vi "CloseConnection.vi"(8 "error in (no error)":errorcluster, 11 "I2COUSBSim in":refnum<class "I2COUSBSim.lvclass">) -> (0 "error out":errorcluster, 1 "Status":string, 3 "I2COUSBSim out":refnum<class "I2COUSBSim.lvclass">)   [LabVIEW 2020, in "I2COUSBSim.lvlib" / "I2COUSBSim.lvclass"]
doc: "Close connection"
uses:
  I2COUSBSim.lvclass
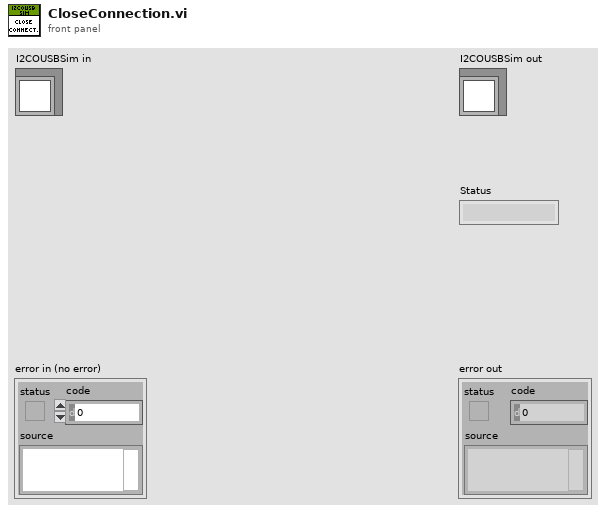
[diagram p1: front panel]
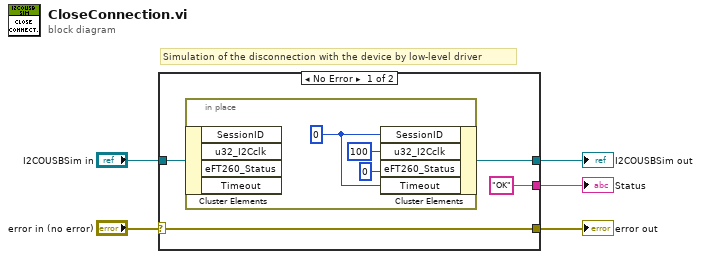
[diagram p0: block diagram]
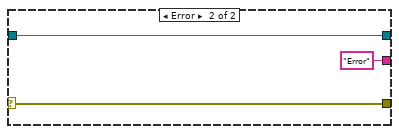
[diagram p2: hidden frame]
diagram:
  # "Simulation of the disconnection with the device by low-level driver"
  n1 = case shown="No Error" "error in (no error)" {
    selector: "error in (no error)" -> [w7 w14]
    tunnel: "I2COUSBSim in" -> [w9 w15]
    tunnel: [w8 w15] -> w4
    tunnel: [w7 w14] -> w2
    tunnel: ["OK" ("Status") "Error" ("Status")] -> w1
    frame No Error {
      n2 = in-place {
        w12 = u32 0 ("SessionID")
        n3 = in-place-cluster #1(w9) -> ()  [unwired: 4 out]
        n4 = in-place-cluster #1("SessionID"=w12, "u32_I2Cclk"=u32 100, "eFT260_Status"=u8 0, "Timeout"=w12) -> (w8:refnum<class "I2COUSBSim.lvclass">)
      }
    }
    frame Error {
    }
  }
  "error out" <- w2
  "I2COUSBSim out" <- w4
  "Status" <- w1
